vi "RT_Main Stop(FGV).vi"(1 "Normal FGV Method":T1, 3 "Stop In":bool) -> (0 "Stop Out":bool)   [LabVIEW 2018]
uses:
  Data Def/RT_Normal FGV Method.ctl
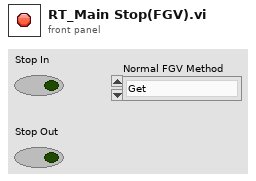
[diagram p1: front panel]
types:
  T1 = typedef "RT_Normal FGV Method.ctl" = enum16{"Get", "Put"}
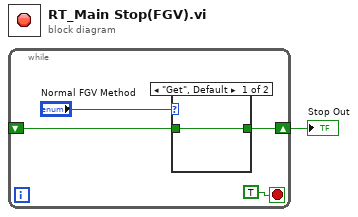
[diagram p0: block diagram]
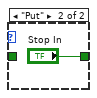
[diagram p2: hidden frame]
diagram:
  n1 = while {
    shift-right: [w3] -> w1
    shift-left: _ -> [w2]
    stop <- TRUE stop-if-true
    n2 = case shown="\"Get\", Default" "Normal FGV Method" {
      tunnel: [w6 "Stop In"] -> w3
      tunnel: w2 -> [w6 _]
      frame "Get", Default {
      }
      frame "Put" {
      }
    }
  }
  "Stop Out" <- w1
